vi "Field Pattern.vi"() -> ()   [LabVIEW 2009]
uses:
  <vilib>/imath/engines/lvmath2/RunTimeEngine/ErrorHandling/NIMS_Finalize Error.vi
  <vilib>/imath/engines/lvmath2/RunTimeEngine/Parser/MC_Version.vi
  <vilib>/imath/engines/lvmath2/RunTimeEngine/Managers/WorkSpace/UID Generator.vi
  <vilib>/imath/engines/lvmath2/RunTimeEngine/NodeEndStatement/NIMS_NodeEndStatement_Output.vi
  <instcachedir>/0/NIMS_NodeEndStatement_Output_B70DDD75627E4997AAE11E9955EDAA25.lvgen/NIMS_NodeEndStatement_Output_B70DDD75627E4997AAE11E9955EDAA25_000.vi
  <vilib>/imath/engines/lvmath2/RunTimeEngine/Managers/SymbolTable/Clear UID.vi
  <vilib>/imath/engines/lvmath2/RunTimeEngine/LocalVariableDefStatement/MC_LocalVariableDefStatement_Display.vi
  <vilib>/imath/engines/lvmath2/RunTimeEngine/RunTimeType/NIMS_RunTimeType_From StrictType (excl LVString).vi
  <vilib>/imath/engines/lvmath2/RunTimeEngine/RangeToken/NIMS_Range.vi
  <instcachedir>/0/NIMS_Range_6D647EC16A744C98B5DE1D649A2D648D.lvgen/NIMS_Range_6D647EC16A744C98B5DE1D649A2D648D_001.vi
  <vilib>/imath/engines/lvmath/Functions/Error Handling/error.ctl
  <vilib>/imath/engines/lvmath/Functions/Error Handling/MergeErrorsWrapper.vi
  <vilib>/imath/engines/lvmath2/RunTimeEngine/VariableToken/NIMS_VariableToken_CondDefined.vi
  <instcachedir>/0/NIMS_VariableToken_CondDefined_5641E79000FB4D628475532441475385.lvgen/NIMS_VariableToken_CondDefined_5641E79000FB4D628475532441475385_001.vi
  <vilib>/imath/engines/lvmath/Functions/Error Handling/MC_Mask_Errors.vi
  <vilib>/imath/engines/lvmath2/RunTimeEngine/BuiltInFunctions/rem/NIMS_rem_no checks.vi
  <instcachedir>/0/NIMS_rem_no checks_4CC9B305AB7E42EF90AFC4973FB32F8D.lvgen/NIMS_rem_no checks_4CC9B305AB7E42EF90AFC4973FB32F8D_000.vi
  <vilib>/imath/engines/lvmath2/RunTimeEngine/BuiltInFunctions/uint32/NIMS_uint32(real).vi
  <instcachedir>/0/NIMS_uint32(real)_FDC83D68D45943DDB8F3F934FF8A712F.lvgen/NIMS_uint32(real)_FDC83D68D45943DDB8F3F934FF8A712F_000.vi
  <vilib>/imath/engines/lvmath2/RunTimeEngine/BuiltInFunctions/double/NIMS_double.vi
  <instcachedir>/0/NIMS_double_2CE444F3CE4146B199A482FE12545E45.lvgen/NIMS_double_2CE444F3CE4146B199A482FE12545E45_000.vi
  <vilib>/imath/engines/lvmath2/RunTimeEngine/BuiltInFunctions/length/NIMS_length(GV).vi
  <instcachedir>/0/NIMS_length(GV)_7D6E94E728E145E68721C53861296D96.lvgen/NIMS_length(GV)_7D6E94E728E145E68721C53861296D96_000.vi
  <instcachedir>/0/NIMS_Range_6D647EC16A744C98B5DE1D649A2D648D.lvgen/NIMS_Range_6D647EC16A744C98B5DE1D649A2D648D_000.vi
  <vilib>/imathl/engines/lvmath/Functions/Error Handling/Create Error.vi
  <vilib>/imath/engines/lvmath2/RunTimeEngine/ReplaceToken/NIMS_Replace - V(S)=S.vi
  <instcachedir>/0/NIMS_Replace - V(S)=S_670A9E0533664C1D848C8E58B3321B6A.lvgen/NIMS_Replace - V(S)=S_670A9E0533664C1D848C8E58B3321B6A_002.vi
  <vilib>/imath/engines/lvmath2/RunTimeEngine/ReplaceToken/NIMS_Replace - Size Check _(_)=S.vi
  <instcachedir>/0/NIMS_Replace - Size Check _(_)=S_8596181D73404097BAB9CBB006194BB0.lvgen/NIMS_Replace - Size Check _(_)=S_8596181D73404097BAB9CBB006194BB0_002.vi
  <vilib>/imath/engines/lvmath2/RunTimeEngine/ReplaceToken/NIMS_Replace - Check Linear.vi
  <instcachedir>/0/NIMS_Replace - Check Linear_9243CBB174894FF6977027453DA6955E.lvgen/NIMS_Replace - Check Linear_9243CBB174894FF6977027453DA6955E_002.vi
  <vilib>/imath/engines/lvmath2/RunTimeEngine/VariableToken/NIMS_VariableToken_CondDefinedDefinedByReplace.vi
  <instcachedir>/0/NIMS_VariableToken_CondDefinedDefinedByReplace_D162CFFC24174562A9FEA619A91E1A56.lvgen/NIMS_VariableToken_CondDefinedDefinedByReplace_D162CFFC24174562A9FEA619A91E1A56_002.vi
  <vilib>/imath/engines/lvmath2/RunTimeEngine/CommandStatement/MC_CommandStatement_break.vi
  <vilib>/imath/engines/lvmath2/RunTimeEngine/ArithmeticOperatorToken/NIMS_ArithmeticOperator_times.vi
  <instcachedir>/0/NIMS_ArithmeticOperator_times_3987BC660D7947CD8628C10658A43225.lvgen/NIMS_ArithmeticOperator_times_3987BC660D7947CD8628C10658A43225_001.vi
  <instcachedir>/0/NIMS_NodeEndStatement_Output_B70DDD75627E4997AAE11E9955EDAA25.lvgen/NIMS_NodeEndStatement_Output_B70DDD75627E4997AAE11E9955EDAA25_001.vi
  <instcachedir>/0/NIMS_ArithmeticOperator_times_3987BC660D7947CD8628C10658A43225.lvgen/NIMS_ArithmeticOperator_times_3987BC660D7947CD8628C10658A43225_000.vi
  <vilib>/imath/engines/lvmath2/RunTimeEngine/VariableToken/Read/NIMS_Get Elements - RV(_) - Check.vi
  <instcachedir>/0/NIMS_Get Elements - RV(_) - Check_60F12861D0564803969A5D0D0D1716CD.lvgen/NIMS_Get Elements - RV(_) - Check_60F12861D0564803969A5D0D0D1716CD_000.vi
  <vilib>/imath/engines/lvmath2/RunTimeEngine/BuiltInFunctions/abs/NIMS_abs(signed).vi
  <instcachedir>/0/NIMS_abs(signed)_C4FCB8E6058B49B797C7C8D53CA5F6EC.lvgen/NIMS_abs(signed)_C4FCB8E6058B49B797C7C8D53CA5F6EC_000.vi
  <instcachedir>/0/NIMS_VariableToken_CondDefined_5641E79000FB4D628475532441475385.lvgen/NIMS_VariableToken_CondDefined_5641E79000FB4D628475532441475385_003.vi
  <instcachedir>/0/NIMS_Replace - V(S)=S_670A9E0533664C1D848C8E58B3321B6A.lvgen/NIMS_Replace - V(S)=S_670A9E0533664C1D848C8E58B3321B6A_001.vi
  <instcachedir>/0/NIMS_Replace - Size Check _(_)=S_8596181D73404097BAB9CBB006194BB0.lvgen/NIMS_Replace - Size Check _(_)=S_8596181D73404097BAB9CBB006194BB0_001.vi
  <instcachedir>/0/NIMS_Replace - Check Linear_9243CBB174894FF6977027453DA6955E.lvgen/NIMS_Replace - Check Linear_9243CBB174894FF6977027453DA6955E_001.vi
  <instcachedir>/0/NIMS_VariableToken_CondDefinedDefinedByReplace_D162CFFC24174562A9FEA619A91E1A56.lvgen/NIMS_VariableToken_CondDefinedDefinedByReplace_D162CFFC24174562A9FEA619A91E1A56_001.vi
  <instcachedir>/0/NIMS_VariableToken_CondDefined_5641E79000FB4D628475532441475385.lvgen/NIMS_VariableToken_CondDefined_5641E79000FB4D628475532441475385_000.vi
  <instcachedir>/0/NIMS_Replace - V(S)=S_670A9E0533664C1D848C8E58B3321B6A.lvgen/NIMS_Replace - V(S)=S_670A9E0533664C1D848C8E58B3321B6A_000.vi
  <instcachedir>/0/NIMS_Replace - Size Check _(_)=S_8596181D73404097BAB9CBB006194BB0.lvgen/NIMS_Replace - Size Check _(_)=S_8596181D73404097BAB9CBB006194BB0_000.vi
  <instcachedir>/0/NIMS_Replace - Check Linear_9243CBB174894FF6977027453DA6955E.lvgen/NIMS_Replace - Check Linear_9243CBB174894FF6977027453DA6955E_000.vi
  <instcachedir>/0/NIMS_VariableToken_CondDefinedDefinedByReplace_D162CFFC24174562A9FEA619A91E1A56.lvgen/NIMS_VariableToken_CondDefinedDefinedByReplace_D162CFFC24174562A9FEA619A91E1A56_000.vi
  <vilib>/gmath/NI_Gmath.lvlib
  <vilib>/imath/engines/lvmath2/RunTimeEngine/Managers/SymbolTable/NIMS_WorkSpace.lvlib
panel:
  in  "?":T1(tab)
  out "XY Graph":cluster{"Y":dbl[], "Y":dbl[]}[](graph)
  out "XY Graph 2":cluster{"Y":dbl[], "Y":dbl[]}[](graph)
  in  "?":enum32{"ATTENUATOR"}(tab)
  out "?":dbl[](graph)
  in  "Set the value of attenuation in dB":dbl(slide) scale=0.0..100.0
  out "?":errorcluster
  in  "HELP FOR ATTENUATOR":bool
  out "error out":errorcluster
  in  "?":enum32{"ISOLATOR"}(tab)
  out "?":dbl[](graph)
  in  "?":bool
  out "?":errorcluster
  in  "HELP FOR ISOLATOR":bool
  out "error out":errorcluster
  in  "?":enum32{"MODULATOR"}(tab)
  in  "Modulating Frequency(KHz)":dbl(slide) scale=0.5..1.5
  out "?":errorcluster
  out "?":dbl[](graph)
  in  "HELP FOR MODULATOR":bool
  out "error out":errorcluster
  in  "?":enum32{"SOURCE"}(tab)
  out "?":dbl[](graph)
  in  "Frequency of carrier wave(GHz)":dbl(slide) scale=8.0..15.0
  in  "Voltage":dbl(knob) scale=0.0..20.0 scale format="%#_10g"
  out "?":errorcluster
  in  "HELP FOR SOURCE":bool
  out "error out":errorcluster
  # "Source"
  # "Tramsmitting and Receiving Antenna"
  # "VSWR meter"
  # "Variable Attenuator"
  # "Coaxial to rectangular adapter"
  # "Connecting waveguide"
  # "Connecting waveguide"
  # "Isolator"
  # "Backward Direction"
  # "Forward direction"
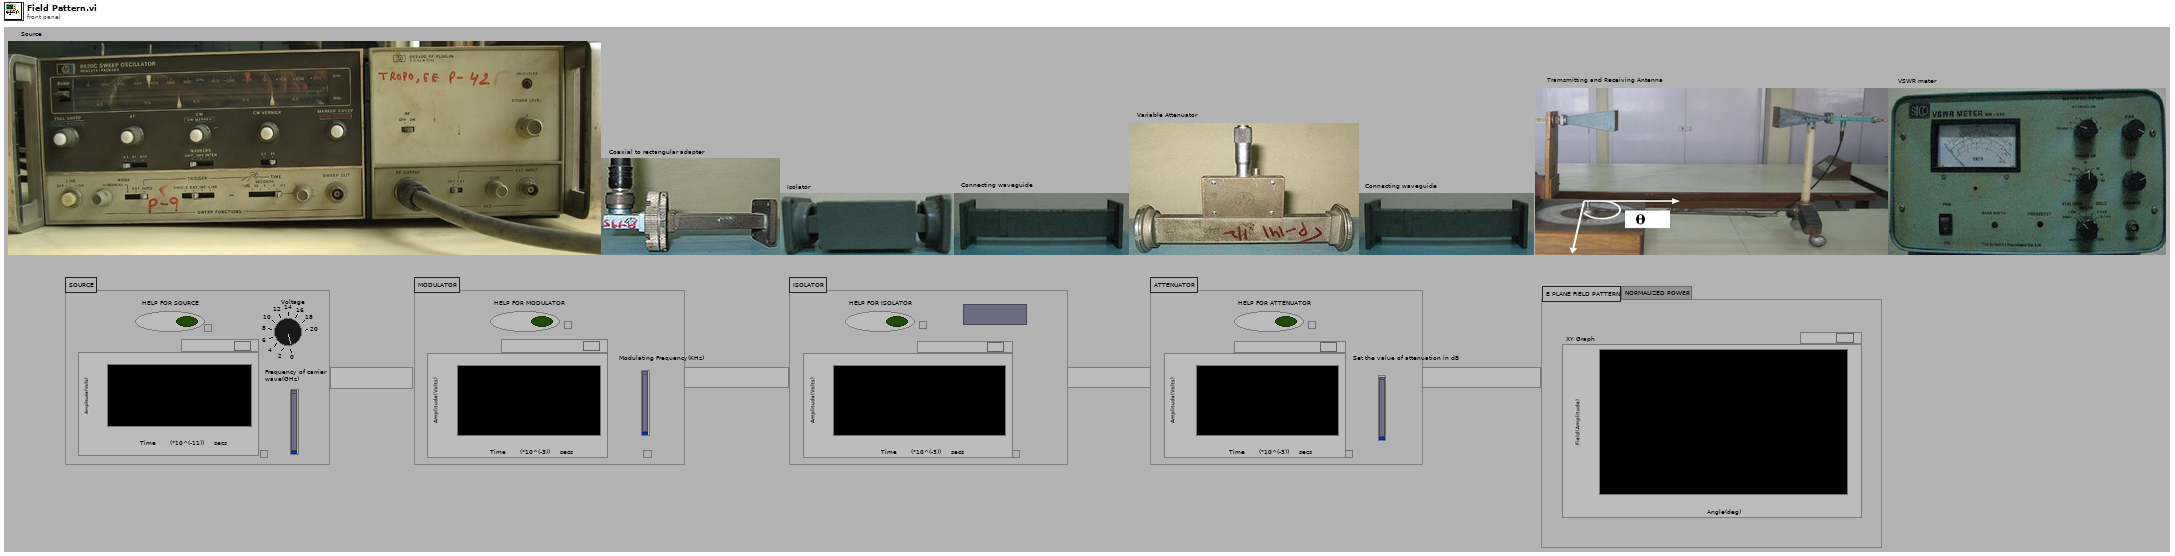
[diagram p1: front panel]
types:
  T1 = enum32{"E PLANE FIELD PATTERN", "NORMALIZED POWER"}
  T2 = typedef "imagedata.ctl" = cluster{"image type":i32, "image depth":i32, "image":u8[], "mask":u8[], "colors":u32[], "Rectangle":cluster{"left":i16, "top":i16, "right":i16, "bottom":i16}}
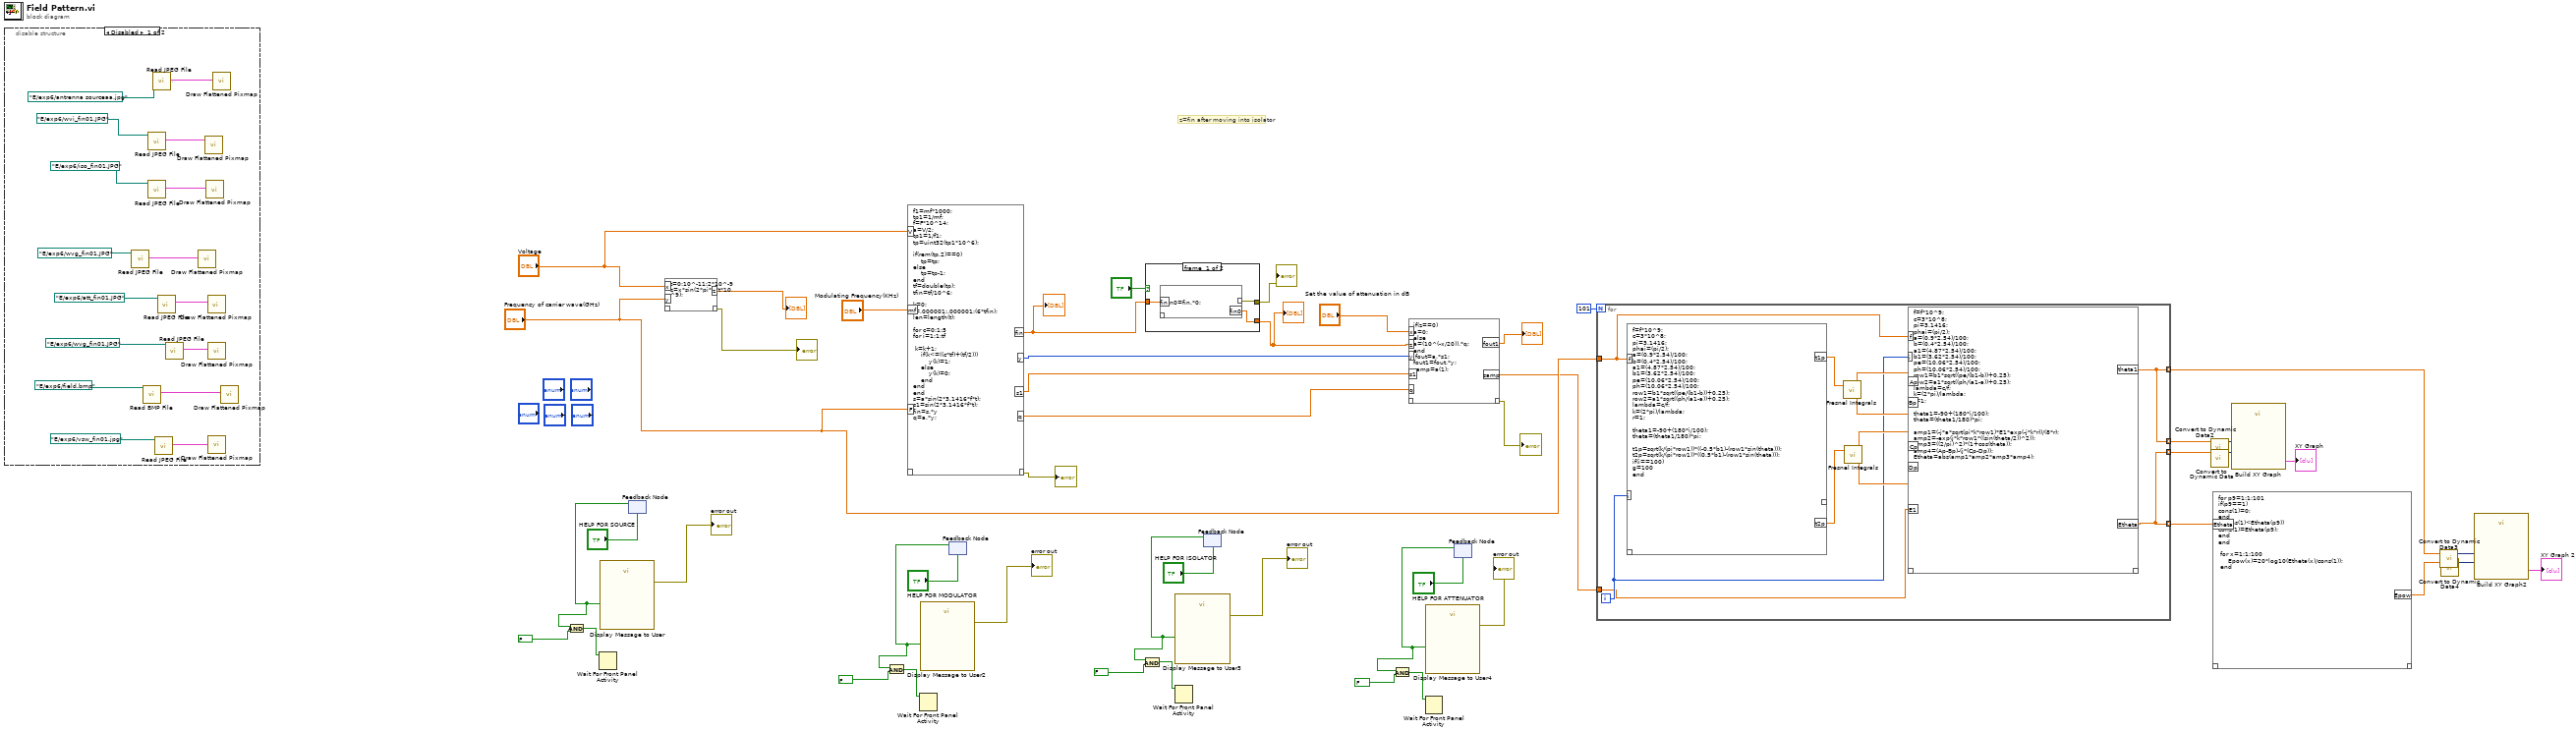
[diagram p0: block diagram]
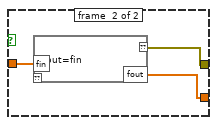
[diagram p3: hidden frame]
diagram:
  # "z=fin after moving into isolator"
  n1 = disable-structure shown="Disabled" {
    frame #0 {
      n2 = call <vilib>:"Read JPEG File.vi"("path to JPEG file"=path "E:/exp6/wvg_fin01.JPG" ("Connecting waveguide")) -> ("image data"=w65:T2)  [unwired: 8 in, 2 out]
      n3 = call <vilib>:"Read BMP File.vi"("path to BMP file"=path "E:/exp6/field.bmp" ("Tx and Rx")) -> ("image data"=w56:T2)  [unwired: 8 in, 2 out]
      n4 = call <vilib>:"Read JPEG File.vi"("path to JPEG file"=path "E:/exp6/wvi_fin01.JPG" ("coaxial rectangular adapter")) -> ("image data"=w67:T2)  [unwired: 8 in, 2 out]
      n5 = call <vilib>:"Read JPEG File.vi"("path to JPEG file"=path "E:/exp6/iso_fin01.JPG" ("Isolator")) -> ("image data"=w55:T2)  [unwired: 8 in, 2 out]
      n6 = call <vilib>:"Read JPEG File.vi"("path to JPEG file"=path "E:/exp6/antrenna sourceaa.jpg" ("source")) -> ("image data"=w69:T2)  [unwired: 8 in, 2 out]
      n7 = call <vilib>:"Read JPEG File.vi"("path to JPEG file"=path "E:/exp6/vsw_fin01.jpg" ("VSWR meter 2")) -> ("image data"=w58:T2)  [unwired: 8 in, 2 out]
      n8 = call <vilib>:"Read JPEG File.vi"("path to JPEG file"=path "E:/exp6/att_fin01.JPG" ("Variable Attenuator 2")) -> ("image data"=w60:T2)  [unwired: 8 in, 2 out]
      n9 = call <vilib>:"Read JPEG File.vi"("path to JPEG file"=path "E:/exp6/wvg_fin01.JPG" ("Connecting Waveguide 3")) -> ("image data"=w62:T2)  [unwired: 8 in, 2 out]
      n10 = call <vilib>:"Draw Flattened Pixmap.vi"("image data"=w65) -> ()  [unwired: 8 in, 1 out]
      n11 = call <vilib>:"Draw Flattened Pixmap.vi"("image data"=w67) -> ()  [unwired: 8 in, 1 out]
      n12 = call <vilib>:"Draw Flattened Pixmap.vi"("image data"=w55) -> ()  [unwired: 8 in, 1 out]
      n13 = call <vilib>:"Draw Flattened Pixmap.vi"("image data"=w60) -> ()  [unwired: 8 in, 1 out]
      n14 = call <vilib>:"Draw Flattened Pixmap.vi"("image data"=w62) -> ()  [unwired: 8 in, 1 out]
      n15 = call <vilib>:"Draw Flattened Pixmap.vi"("image data"=w58) -> ()  [unwired: 8 in, 1 out]
      n16 = call <vilib>:"Draw Flattened Pixmap.vi"("image data"=w69) -> ()  [unwired: 8 in, 1 out]
      n17 = call <vilib>:"Draw Flattened Pixmap.vi"("image data"=w56) -> ()  [unwired: 8 in, 1 out]
    }
    frame #1 {
    }
  }
  n18 = feedback #1("HELP FOR SOURCE") -> (w48:bool)
  n19 = And(x=w48, y=FALSE) -> (x .and. y?=w46:bool)
  n20 = Wait For Front Panel Activity(3:w46) -> ()  [unwired: 3 out]
  n21 = call "Display Message to User"("Enable"=w48) -> ("error out"=→"error out":errorcluster, "CLOSE"=w50:bool)  [unwired: 2 in, 7 out]
  n22 = mathscript code="t=0:10^-11:2*10^-9\nz=x*sin(2*pi*y*t*10^9);"("x"="Voltage", "y"="Frequency of carrier wave(GHz)") -> ("??"=→"?":errorcluster, "z"=→"?":dbl[])  [unwired: 1 in]
  n23 = mathscript code="f1=mf*1000;\ntp1=1/mf;\nf=F*10^14;\na=V/2;\ntp1=1/f1;\ntp=uint32(tp1*10^6);\n\nif(rem(tp,2)==0)\n    tp=tp;\nelse\n    tp=tp-1;\nend\ntf=double(tp);\ntfin=tf/10^6;\n\nk=0;\nt=.000001:.000001:(6*tfin);\nlen=length(t);\n\nfor c=0:1:5\nfor i=1:1:tf\n  \n k=k+1;\n    if(k<=((c*tf)+(tf/2)))\n        y(k)=1;\n    else\n        y(k)=0;\n    end\nend\nend\ns=a*sin(2*3.1416*f*t);\ns1=sin(2*3.1416*f*t);\nfin=s.*y\nq=a.*y;"("V"="Voltage", "mf"="Modulating Frequency(KHz)", "F"="Frequency of carrier wave(GHz)") -> ("??"=→"?":errorcluster, "y"=w5:i32[], "s1"=w12:dbl[], "q"=w11:dbl[], "fin"=w4:dbl[])  [unwired: 1 in]
  "?" <- w4
  n24 = feedback #2("HELP FOR MODULATOR") -> (w42:bool)
  n25 = And(x=w42, y=FALSE) -> (x .and. y?=w40:bool)
  n26 = Wait For Front Panel Activity(3:w40) -> ()  [unwired: 3 out]
  n27 = call "Display Message to User2"("Enable"=w42) -> ("error out"=→"error out":errorcluster, "CLOSE"=w44:bool)  [unwired: 2 in, 7 out]
  n28 = case shown="True" "?" {
    tunnel: [w71 w92] -> w3
    tunnel: [w72 w93] -> w52
    tunnel: w4 -> [w70 w91]
    frame #0 {
      n29 = mathscript code="fin0=fin.*0;"("fin"=w70) -> ("??"=w72:errorcluster, "fin0"=w71:dbl[])  [unwired: 1 in]
    }
    frame #1 {
      n30 = mathscript code="fout=fin"("fin"=w91) -> ("??"=w93:errorcluster, "fout"=w92:dbl[])  [unwired: 1 in]
    }
  }
  "?" <- w3
  "?" <- w52
  n31 = feedback #3("HELP FOR ISOLATOR") -> (w36:bool)
  n32 = And(x=w36, y=FALSE) -> (x .and. y?=w34:bool)
  n33 = Wait For Front Panel Activity(3:w34) -> ()  [unwired: 3 out]
  n34 = call "Display Message to User3"("Enable"=w36) -> ("error out"=→"error out":errorcluster, "CLOSE"=w38:bool)  [unwired: 2 in, 7 out]
  n35 = mathscript code="if(z==0)\na=0; \nelse\na=(10^(-x/20)).*q;\nend\n fout=a.*s1;\nfout1=fout.*y;\nsamp=a(1);"("x"="Set the value of attenuation in dB", "z"=w3, "y"=w5, "s1"=w12, "q"=w11) -> ("??"=→"?":errorcluster, "fout1"=→"?":dbl[], "samp"=w6:dbl)  [unwired: 1 in]
  n36 = feedback #4("HELP FOR ATTENUATOR") -> (w30:bool)
  n37 = And(x=w30, y=FALSE) -> (x .and. y?=w28:bool)
  n38 = Wait For Front Panel Activity(3:w28) -> ()  [unwired: 3 out]
  n39 = call "Display Message to User4"("Enable"=w30) -> ("error out"=→"error out":errorcluster, "CLOSE"=w32:bool)  [unwired: 2 in, 7 out]
  n40 = for {
    N: 101 -> [_]
    tunnel: "Frequency of carrier wave(GHz)" -> [w129]
    tunnel: [w126] -> w24 mode=indexing
    tunnel: [w128] -> w22 mode=indexing
    tunnel: [w126] -> w20 mode=indexing
    tunnel: [w128] -> w19 mode=indexing
    tunnel: w6 -> [w127]
    i -> [w130]
    n41 = mathscript code="f=f*10^9;\nc=3*10^8;\npi=3.1416;\nphai=(pi/2);\na=(0.9*2.54)/100;\nb=(0.4*2.54)/100;\na1=(4.87*2.54)/100;\nb1=(3.62*2.54)/100;\npe=(10.06*2.54)/100;\nph=(10.06*2.54)/100;\nrow1=b1*sqrt((pe/(b1-b))+0.25);\nrow2=a1*sqrt((ph/(a1-a))+0.25);\nlambda=c/f;\nk=(2*pi)/lambda;\nr=1;\n\ntheta1=-90+(180*i/100);\ntheta=(theta1/180)*pi;\n   \nt1p=sqrt(k/(pi*row1))*((-0.5*b1)-(row1*sin(theta)));\nt2p=sqrt(k/(pi*row1))*((0.5*b1)-(row1*sin(theta)));\nif(i==100)\ng=100\nend"("i"=w130, "f"=w129) -> ("t1p"=w136:dbl, "t2p"=w135:dbl)  [unwired: 2 out]
    n42 = call <vilib>:"Fresnel Integrals.vi"("x"=w136) -> ("S(x)"=w131:dbl, "C(x)"=w133:dbl)  [unwired: 1 out]
    n43 = call <vilib>:"Fresnel Integrals.vi"("x"=w135) -> ("S(x)"=w132:dbl, "C(x)"=w134:dbl)  [unwired: 1 out]
    n44 = mathscript code="f=f*10^9;\nc=3*10^8;\npi=3.1416;\nphai=(pi/2);\na=(0.9*2.54)/100;\nb=(0.4*2.54)/100;\na1=(4.87*2.54)/100;\nb1=(3.62*2.54)/100;\npe=(10.06*2.54)/100;\nph=(10.06*2.54)/100;\nrow1=b1*sqrt((pe/(b1-b))+0.25);\nrow2=a1*sqrt((ph/(a1-a))+0.25);\nlambda=c/f;\nk=(2*pi)/lambda;\nr=1;\n \ntheta1=-90+(180*i/100);\ntheta=(theta1/180)*pi;\n    \namp1=(-j*a*sqrt(pi*k*row1)*E1*exp(-j*k*r))/(8*r);\namp2=-exp(j*k*row1*((sin(theta/2))^2));\namp3=((2/pi)^2)*(1+cos(theta));\namp4=(Ap-Bp)-(j*(Cp-Dp));\nEtheta=abs(amp1*amp2*amp3*amp4);"("Ap"=w134, "Bp"=w133, "Cp"=w132, "Dp"=w131, "i"=w130, "E1"=w127, "f"=w129) -> ("Etheta"=w126:dbl, "theta1"=w128:dbl)  [unwired: 2 out]
  }
  n45 = call "Convert to Dynamic Data2"("Array"=w22) -> ("Dynamic Data Type"=w21:dynamicdata)  [unwired: 3 out]
  n46 = call "Convert to Dynamic Data"("Array"=w24) -> ("Dynamic Data Type"=w23:dynamicdata)  [unwired: 3 out]
  n47 = mathscript code="for p9=1:1:101\nif(p9==1)\ncons(1)=0;\nend\nif(cons(1)<Etheta(p9))\ncons(1)=Etheta(p9);\nend\nend\n\n for x=1:1:100\n     Epow(x)=20*log10(Etheta(x)/cons(1));\n end"("Etheta"=w20) -> ("Epow"=w17:dbl[])  [unwired: 2 out]
  n48 = call "Build XY Graph"("Y Input"=w23, "X Input"=w21) -> ("XY Graph"=→"XY Graph":cluster{"Y":dbl[], "Y":dbl[]}[])  [unwired: 3 in, 6 out]
  n49 = call "Convert to Dynamic Data3"("Array"=w19) -> ("Dynamic Data Type"=w18:dynamicdata)  [unwired: 3 out]
  n50 = call "Convert to Dynamic Data4"("Array"=w17) -> ("Dynamic Data Type"=w16:dynamicdata)  [unwired: 3 out]
  n51 = call "Build XY Graph2"("Y Input"=w16, "X Input"=w18) -> ("XY Graph"=→"XY Graph 2":cluster{"Y":dbl[], "Y":dbl[]}[])  [unwired: 3 in, 6 out]
